vi "Test set value on undefined cell.vi"(11 "Test Case In":refnum<class "Test Cases.lvclass">) -> (0 "error out":errorcluster, 3 "Test Case Out":refnum<class "Test Cases.lvclass">)   [LabVIEW 2023, in "Test Cases.lvclass"]
uses:
  Test Cases.lvclass
  C:/Program Files/National Instruments/LabVIEW 2025/vi.lib/Astemes/LUnit/Test Case.lvclass
  D:/git/Sourcegrid-LabVIEW/dll/SourceGrid.dll
  dll/SourceGrid.dll
  source/Grid/SourceGrid.lvclass
  <vilib>/Astemes/LUnit/Test Case.lvclass/Test Case.ctl
  <vilib>/Astemes/LUnit/Append Fail Result.vi
  <vilib>/Astemes/LUnit/Append Pass Result.vi
  <vilib>/Astemes/LUnit/Run In UI.vi
  source/Grid/Set Column Default Width.vi
  <vilib>/Astemes/LUnit/Test Case.lvclass
panel:
  in  "stop":bool
  in  "Grid Container":refnum<k24>(container)
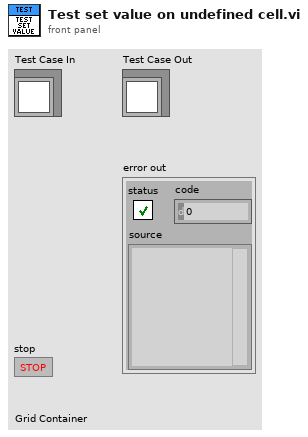
[diagram p1: front panel]
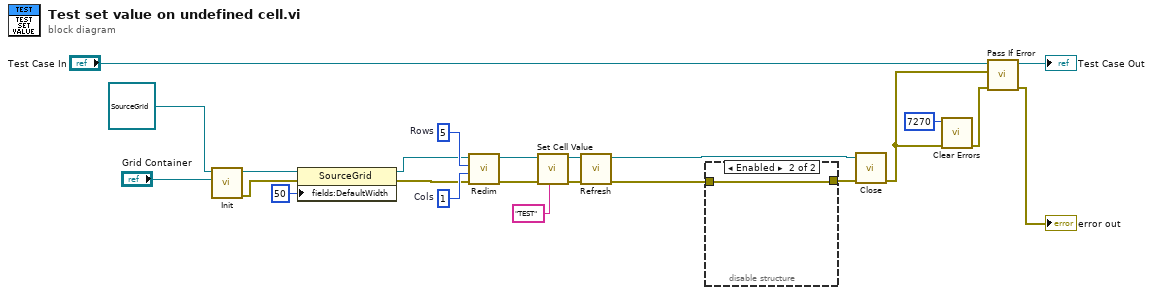
[diagram p0: block diagram]
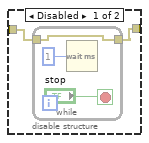
[diagram p2: hidden frame]
diagram:
  w19 = 1  # Cols
  w20 = 5  # Rows
  n1 = call-dynamic "Init.vi"("Sourcegrid Container"="Grid Container", "Grid in"=refnum<class "SourceGrid.lvclass"> refnum) -> ("error out"=w10:errorcluster, "Grid out"=w17:refnum<class "SourceGrid.lvclass">)  [unwired: 8 in]
  n2 = property class="SourceGrid"(reference=w17, error in=w10, "fields:DefaultWidth"=50 ("DefaultWidth")) -> (reference out=w16:refnum<class "SourceGrid.lvclass">, error out=w15:errorcluster)
  n3 = call "Redim.vi"("error in"=w15, "Columns"=w19, "Rows"=w20, "Sourcegrid in"=w16) -> ("error out"=w8:errorcluster, "Sourcegrid out"=w13:refnum<class "SourceGrid.lvclass">)  [unwired: 6 in]
  n4 = call "Set Cell Value.vi"("Value"="TEST", "error in"=w8, "SourceGrid in"=w13) -> ("error out"=w7:errorcluster, "SourceGrid out"=w6:refnum<class "SourceGrid.lvclass">)  [unwired: 7 in]
  n5 = call "Refresh.vi"("error in"=w7, "SourceGrid in"=w6) -> ("error out"=w5:errorcluster, "SourceGrid out"=w11:refnum<class "SourceGrid.lvclass">)  [unwired: 8 in]
  n6 = disable-structure shown="Enabled" {
    disable-tunnel: w5 -> [w25 w29]
    disable-tunnel: [w24 w29] -> w9
    frame Disabled {
      n7 = while {
        tunnel: w25 -> [w26]
        tunnel: [w26] -> w24
        stop <- "stop" stop-if-true
        n8 = Wait (ms)(milliseconds to wait=u32 1) -> ()  [unwired: 1 out]
      }
    }
    frame Enabled {
    }
  }
  n9 = call-dynamic "Close.vi"("error in"=w9, "Sourcegrid in"=w11) -> ("error out"=w2:errorcluster)  [unwired: 8 in, 1 out]
  n10 = call <vilib>:"Clear Errors.vi"("error in (no error)"=w2, "specific error code to clear (0: all)"=7270) -> ("error out"=w3:errorcluster)  [unwired: 4 in, 1 out]
  n11 = call <vilib>:"Pass If Error.vi"("error in (no error)"=w3, "Assert error"=w2, "LUnit Test Case In"="Test Case In") -> ("error out"=→"error out":errorcluster, "LUnit Test Case Out"=→"Test Case Out":refnum<class "Test Cases.lvclass">)  [unwired: 7 in]
